vi "CallVI.vi"(0 "VI引用":refnum<vi>, 7 "状态":T1(ring)=enum."Standard", 11 "错误输入":errorcluster) -> (4 "VI引用OUT":refnum<vi>, 15 "错误输出":errorcluster)   [LabVIEW 2020]
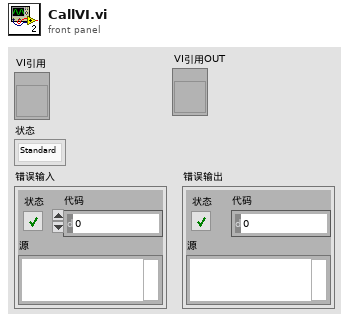
[diagram p1: front panel]
types:
  T1 = enum32{"Invalid", "Standard", "Closed", "Hidden", "Minimized", "Maximized"}
  T2 = enum32{"Bad", "Idle", "Run top level", "Running"}
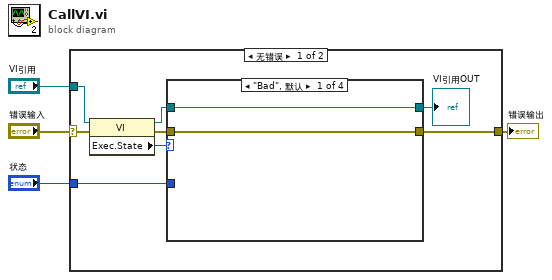
[diagram p0: block diagram]
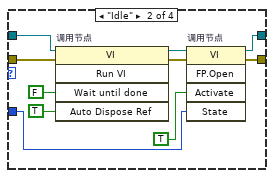
[diagram p2: hidden frame]
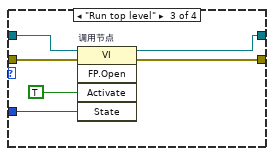
[diagram p3: hidden frame]
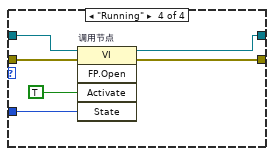
[diagram p4: hidden frame]
diagram:
  n1 = case shown="无错误" "错误输入" {
    selector: "错误输入" -> [w7 w37]
    tunnel: "状态" -> [w10 _]
    tunnel: "VI引用" -> [w9 _]
    tunnel: [w6 w37] -> w1
    frame No Error {
      n2 = property class="VI"(reference=w9, error in=w7) -> (reference out=w11:refnum<vi>, error out=w8:errorcluster, "Exec.State"=w12:T2)
      n3 = case shown="\"Bad\", 默认" w12 {
        tunnel: w11 -> [w13 w24 w30 w36]
        tunnel: w10 -> [_ w21 w29 w35]
        tunnel: w8 -> [w14 w19 w27 w33]
        tunnel: [w14 w17 w26 w32] -> w6
        tunnel: [w13 w16 w25 w31] -> w5
        frame "Bad", Default {
        }
        frame "Idle" {
          n4 = invoke on="调用节点" class="VI" method="Run VI"(reference=w24, error in=w19, "Wait until done"=FALSE ("结束前等待"), "Auto Dispose Ref"=TRUE ("自动销毁引用")) -> (reference out=w23:refnum<vi>, error out=w18:errorcluster)  [unwired: 1 in, 3 out]
          n5 = invoke on="调用节点" class="VI" method="FP.Open"(reference=w23, error in=w18, "Activate"=TRUE ("激活？"), "State"=w21) -> (reference out=w16:refnum<vi>, error out=w17:errorcluster)  [unwired: 1 in, 3 out]
        }
        frame "Run top level" {
          n6 = invoke on="调用节点" class="VI" method="FP.Open"(reference=w30, error in=w27, "Activate"=TRUE ("激活？"), "State"=w29) -> (reference out=w25:refnum<vi>, error out=w26:errorcluster)  [unwired: 1 in, 3 out]
        }
        frame "Running" {
          n7 = invoke on="调用节点" class="VI" method="FP.Open"(reference=w36, error in=w33, "Activate"=TRUE ("激活？"), "State"=w35) -> (reference out=w31:refnum<vi>, error out=w32:errorcluster)  [unwired: 1 in, 3 out]
        }
      }
      "VI引用OUT" <- w5
    }
    frame Error {
    }
  }
  "错误输出" <- w1
